vi "Create.vi"(8 "error in (no error)":errorcluster, 9 "Outputs":string[](array[string]), 10 "Inputs":string[](array[string])) -> (0 "error out":errorcluster, 3 "Conjunction":refnum<class "Conjunction.lvclass">)   [LabVIEW 2021, in "Conjunction.lvclass"]
uses:
  Conjunction.lvclass
  Conjunction.lvclass/Conjunction.ctl
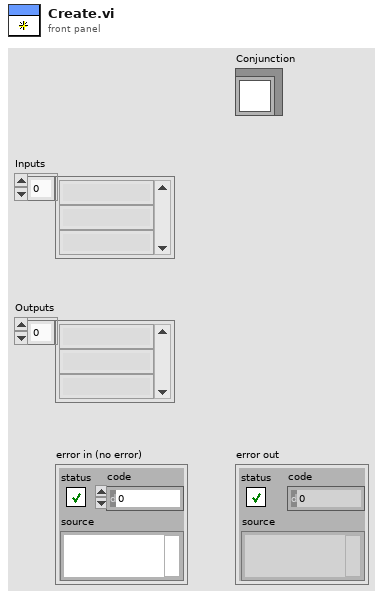
[diagram p1: front panel]
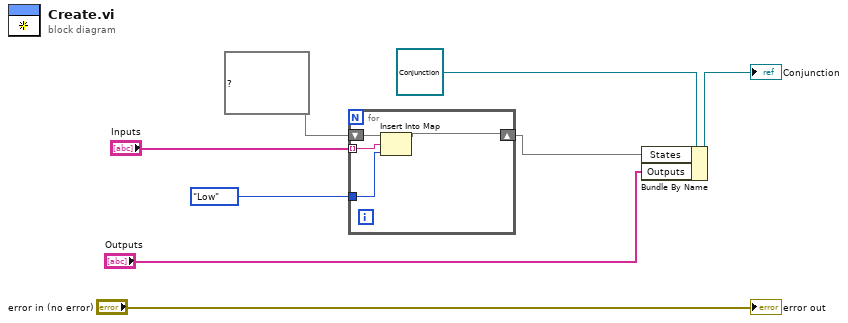
[diagram p0: block diagram]
diagram:
  n1 = for {
    shift-right: [w11] -> w2
    shift-left: map{string, enum16{"Low", "High"}} {} ("map") -> [w12]
    tunnel: "Inputs" -> [w10] mode=indexing
    tunnel: enum16{"Low", "High"}."Low" ("Pulse Out") -> [w9]
    n2 = Insert Into Map(map in=w12, key=w10, value=w9) -> (map out=w11:map{string, enum16{"Low", "High"}})  [unwired: 2 out]
  }
  n3 = Bundle By Name(cluster=refnum<class "Conjunction.lvclass"> refnum ("Conjunction"), "States"=w2, "Outputs"="Outputs") -> (→"Conjunction":refnum<class "Conjunction.lvclass">)
  "error out" <- "error in (no error)"
